vi "Start DAQ.vi"(8 "error in (no error)":errorcluster, 11 "RFSA DAQ in":refnum<class "RFSA DAQ.lvclass">) -> (0 "error out":errorcluster, 3 "RFSA DAQ out":refnum<class "RFSA DAQ.lvclass">)   [LabVIEW 2020, in "RFSA DAQ.lvlib" / "RFSA DAQ.lvclass"]
uses:
  RFSA DAQ.lvclass
  Helper Loop Message.ctl
  Helper Loop Type.ctl
  RFSA DAQ.lvclass/RFSA DAQ.ctl
  DAQ Interface/DAQ Interface/DAQ Interface.lvclass
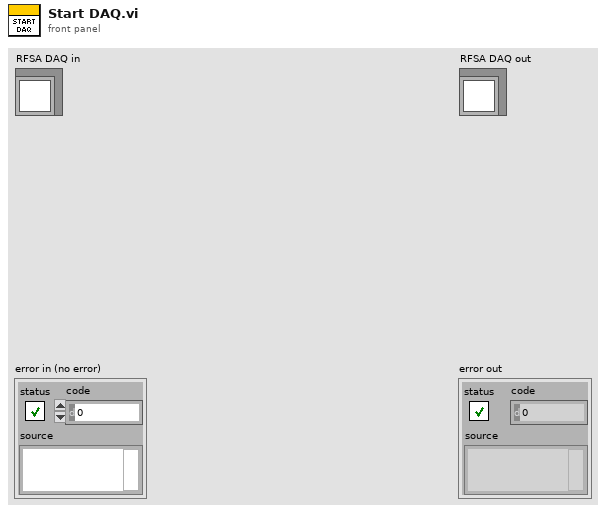
[diagram p1: front panel]
types:
  T1 = typedef "RFSA DAQ.lvlib/RFSA DAQ.lvclass/Helper Loop Message.ctl" = cluster{"Type":T2, "Payload":variant}
  T2 = typedef "RFSA DAQ.lvlib/RFSA DAQ.lvclass/Helper Loop Type.ctl" = enum16{"Configure", "Start", "Do", "Stop", "Clean", "Close"}
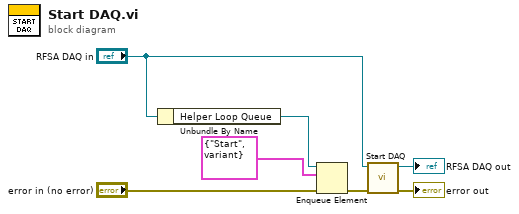
[diagram p0: block diagram]
diagram:
  n1 = Unbundle By Name("RFSA DAQ in") -> ("Helper Loop Queue"=w5:refnum<queue>)
  n2 = Enqueue Element(queue=w5, element=T1 {"Type"=enum."Start", "Payload"=variant}, error in (no error)="error in (no error)") -> (error out=w2:errorcluster)  [unwired: 1 in, 2 out]
  n3 = call-parent "Start DAQ.vi"("error in (no error)"=w2, "DAQ Interface in"="RFSA DAQ in") -> ("error out"=→"error out":errorcluster, "DAQ Interface out"=→"RFSA DAQ out":refnum<class "RFSA DAQ.lvclass">)  [unwired: 8 in]
